vi "GUILib.simple numeric show increment.vi"(0 "ctlRef":refnum<vi>, 2 "show":bool, 5 "error in (no error)":errorcluster) -> (14 "ctlRef dup":refnum<vi>, 19 "error out":errorcluster)   [LabVIEW 2012, in "GUILib.lvlib"]
doc: "shows/hides the increment field for a specific type of control"
uses:
  GUILib.lvlib
panel:
  in  "numericType":dbl
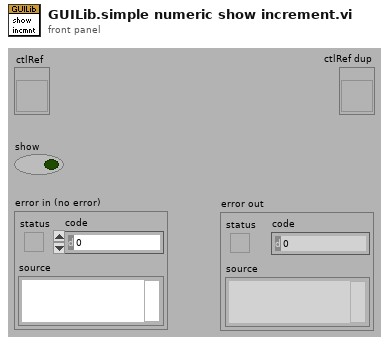
[diagram p1: front panel]
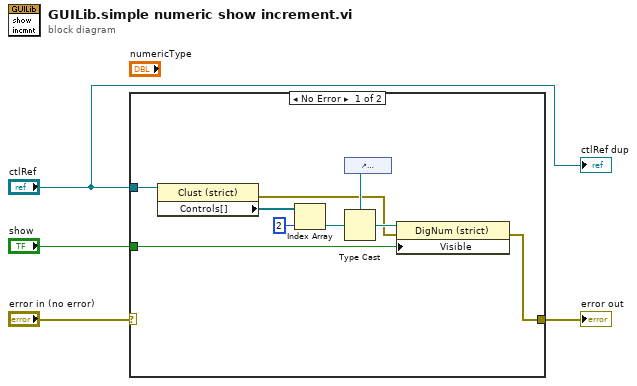
[diagram p0: block diagram]
diagram:
  n1 = case shown="No Error" "error in (no error)" {
    selector: "error in (no error)" -> [_ w14]
    tunnel: "show" -> [w13 _]
    tunnel: "ctlRef" -> [w5 _]
    tunnel: [w6 w14] -> w2
    frame No Error {
      n2 = property class="Clust (strict)"(reference=w5) -> (error out=w7:errorcluster, "Controls[]"=w9:refnum<vi>[])  [unwired: 1 in, 1 out]
      n3 = Index Array(array=w9, index=2) -> (element=w11:refnum<vi>)
      n4 = control-ref of="numericType"() -> (w8:refnum<vi>)
      n5 = Type Cast(type=w8, x=w11) -> (*(type *) &x=w12:refnum<vi>)
      n6 = property class="DigNum (strict)"(reference=w12, error in=w7, "Visible"=w13) -> (error out=w6:errorcluster)  [unwired: 1 out]
    }
    frame Error {
    }
  }
  "error out" <- w2
  "ctlRef dup" <- "ctlRef"
